vi "LauftextTempHum.vi"(1 "Intensity 0-100":dbl(knob) min=0.0 max=100.0 step=1.0 scale=0.0..100.0, 3 "VISA resource name":refnum<visa-resource-name>) -> (0 "VISA resource name 2":refnum<visa-resource-name>)   [LabVIEW 2021]
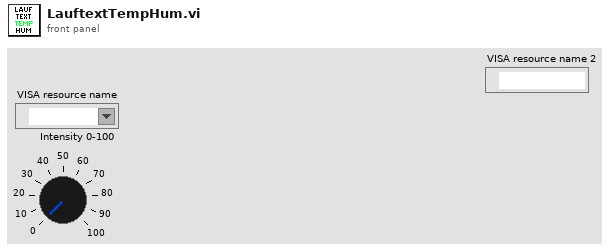
[diagram p1: front panel]
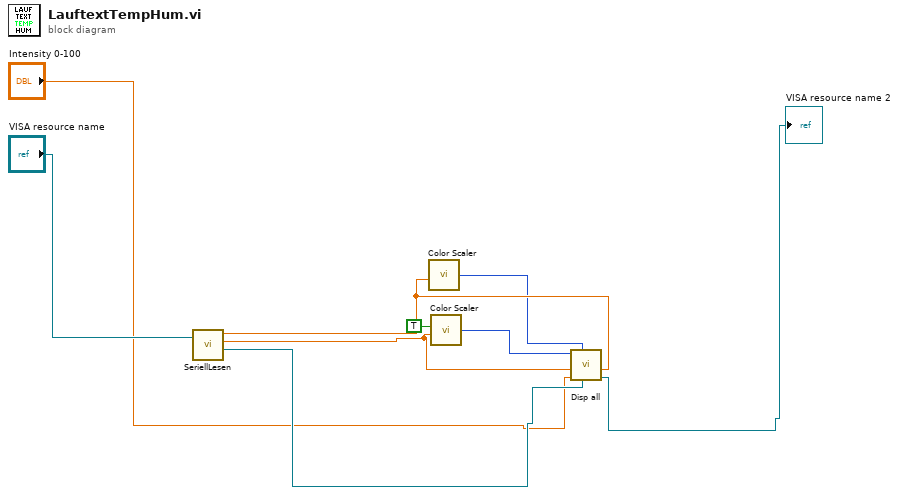
[diagram p0: block diagram]
diagram:
  n1 = call "SeriellLesen.vi"("VISA resource name"="VISA resource name") -> ("Temperatur"=w3:dbl, "Humidity"=w4:dbl, "VISA resource name 2"=w7:refnum<visa-resource-name>)  [unwired: 1 in, 1 out]
  n2 = call "Color Scaler.vi"("Input"=w3) -> ("Output Color"=w2:u32)  [unwired: 5 in]
  n3 = call "Color Scaler.vi"("Input"=w4, "Boolean (False =Temp;True=hum)"=TRUE) -> ("Output Color"=w1:u32)  [unwired: 4 in]
  n4 = call "Disp all.vi"("Temp"=w3, "VISA resource name"=w7, "Temp Colour"=w2, "Intensity 0-100"="Intensity 0-100", "Hum"=w4, "Hum Colour"=w1) -> ("VISA resource name 2"=→"VISA resource name 2":refnum<visa-resource-name>)  [unwired: 3 in]
